vi "Get Array Values (String[]).vi"(8 "error in (no error)":errorcluster, 11 "JSON Value in":refnum<class "JSON Value.lvclass">) -> (0 "error out":errorcluster, 3 "values":string[](array[string]))   [LabVIEW 2017, in "JSON Value.lvclass"]
doc: "Returns the element type of each element in a JSON Array. If all elements are of the same type, single type is true."
uses:
  JSON Value.lvclass
  JSON Types.ctl
  subVIs/Errors.ctl
  Read Value/Read value (String).vi
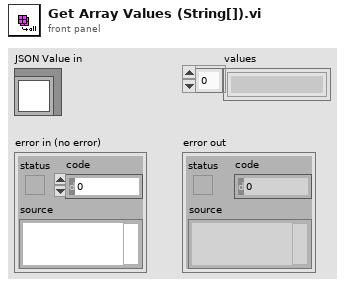
[diagram p1: front panel]
types:
  T1 = typedef "JSON Value.lvclass/JSON Types.ctl" = enum16{"String", "Numeric", "Boolean", "NULL", "Object", "Array"}
  T2 = typedef "JSON Value.lvclass/Errors.ctl" = enum16{"No key", "Key path type", "Array OOB", "Type Mismatch", "Invalid Token"}
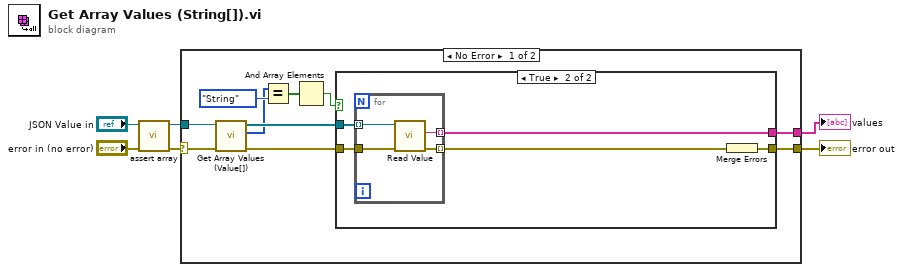
[diagram p0: block diagram]
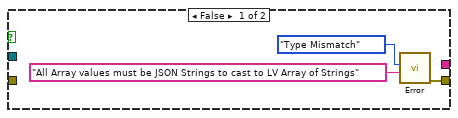
[diagram p2: hidden frame]
diagram:
  n1 = call "assert array.vi"("error in (no error)"="error in (no error)", "JSON Value in"="JSON Value in") -> ("error out"=w3:errorcluster, "JSON Value out"=w1:refnum<class "JSON Value.lvclass">)  [unwired: 8 in]
  n2 = case shown="No Error" w3 {
    selector: w3 -> [w15 w29]
    tunnel: w1 -> [w16 _]
    tunnel: [w13 w29] -> w5
    tunnel: [w11 _] -> w4
    frame No Error {
      n3 = call "Get Array Values (Value[]).vi"("error in (no error)"=w15, "JSON Value in"=w16) -> ("error out"=w10:errorcluster, "types"=w9:T1[], "values"=w14:refnum<class "JSON Value.lvclass">[])  [unwired: 6 in, 1 out]
      n4 = Equal?(x=w9, y=JSON_Types."String") -> (x = y?=w8:bool[])
      n5 = And Array Elements(Boolean array=w8) -> (logical AND=w7:bool)
      n6 = case shown="True" w7 {
        tunnel: w14 -> [_ w24]
        tunnel: [w17 w20] -> w13
        tunnel: [_ w23] -> w11
        tunnel: w10 -> [_ w21]
        frame False {
          n7 = call "Error.vi"("Data"="All Array values must be JSON Strings to cast to LV Array of Strings", 9:Errors."Type Mismatch") -> ("error out"=w17:errorcluster)  [unwired: 8 in]
        }
        frame True {
          n8 = for {
            tunnel: w24 -> [w25] mode=indexing
            tunnel: [w28] -> w23 mode=indexing
            tunnel: [w27] -> w22 mode=indexing
            tunnel: w21 -> [w26]
            n9 = call-poly "Read Value.vi"("error in (no error)"=w26, "JSON String in"=w25) -> ("error out"=w27:errorcluster, "value"=w28:string)  [unwired: 7 in, 1 out]
          }
          n10 = Merge Errors(w22) -> (w20:errorcluster)
        }
      }
    }
    frame Error {
    }
  }
  "error out" <- w5
  "values" <- w4
